vi "例6-4.vi"() -> ()   [LabVIEW 2019]
uses:
  <vilib>/measure/NI_MAPro.lvlib
panel:
  out "实际单频信号频率":dbl[](array[numeric])
  in  "采样信息":cluster{"采样频率":dbl, "采样点数":dbl}={"采样频率"=1000.0, "采样点数"=1000.0}
  in  "初始相位":dbl[](array[numeric])
  in  "幅值":dbl[](array[numeric]) format="%02_2g"
  in  "频率":dbl[](array[numeric])
  out "波形图":waveform(dbl)(graph)
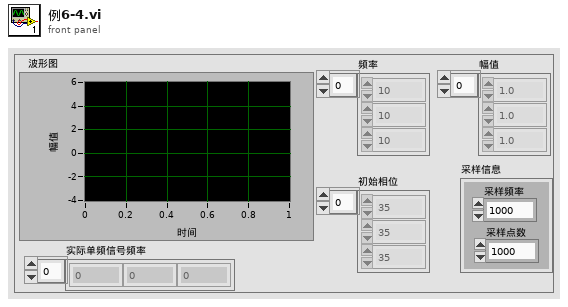
[diagram p1: front panel]
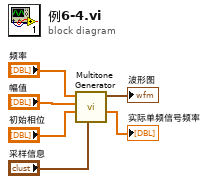
[diagram p0: block diagram]
diagram:
  n1 = call <vilib>:"Multitone Generator.vi"("sampling info"="采样信息", "tone phases"="初始相位", "tone amplitudes"="幅值", "tone frequencies"="频率") -> ("actual tone frequencies"=→"实际单频信号频率":dbl[], "signal out"=→"波形图":waveform(dbl))  [unwired: 4 in, 2 out]
